vi "AMZ_S3_AUTH_Create HTTP Handle.vi"(4 "Use HTTPS?":bool, 6 "HTTP-Verb":string(combo)="GET", 7 "Redirect endpoint":string, 8 "error in (no error)":errorcluster, 9 "Bucket":string, 10 "Path and query string":string, 11 "Headers":T1[](array[typedef])) -> (0 "error out":errorcluster, 2 "URL":string, 3 "client handle out":T2)   [LabVIEW 2015, in "LV Interface for Amazon S3.lvlib"]
doc: "Create an HTTP Client Handle to Amazon AWS. The handle will hold the necessary Authorozation header which is calculated from many parts and signed with the user's SecretKey."
uses:
  LV Interface for Amazon S3.lvlib
  <vilib>/httpClient/ClientHandle.ctl
  Typedefs/AMZ_S3_HTTP Header-Value pair.ctl
  <vilib>/httpClient/LabVIEWHTTPClient.lvlib
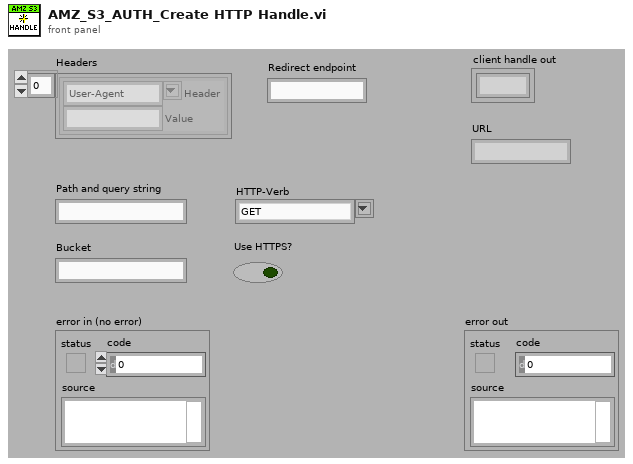
[diagram p1: front panel]
types:
  T1 = typedef "LV Interface for Amazon S3.lvlib/AMZ_S3_HTTP Header-Value pair.ctl" = cluster{"Header":string, "Value":string}
  T2 = typedef "LabVIEWHTTPClient.lvlib/ClientHandle.ctl" = refnum<k1>
  T3 = typedef "LV Interface for Amazon S3.lvlib/AMZ_S3_AWS Credentials.ctl" = cluster{"Access Key":string, "Secret Key":string}
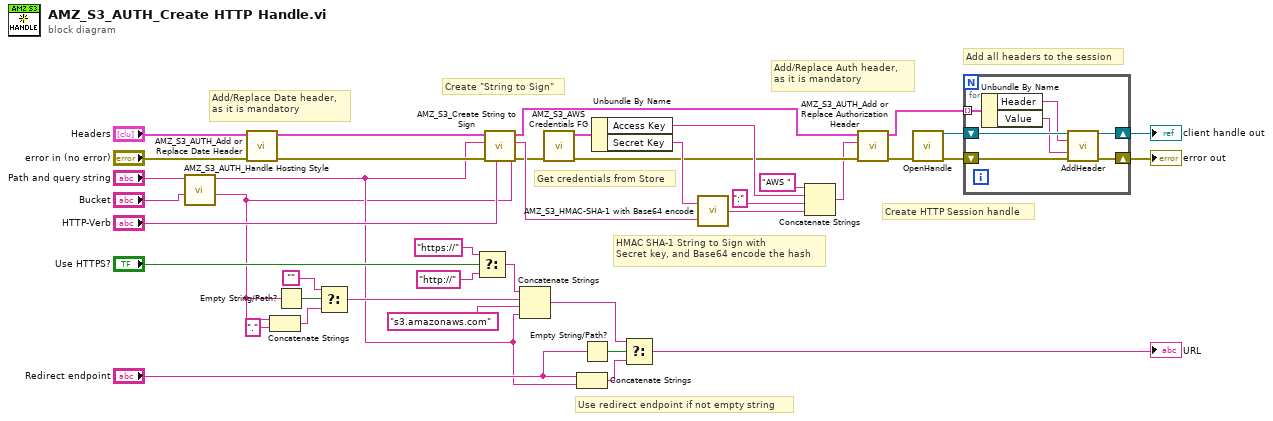
[diagram p0: block diagram]
diagram:
  # "Add all headers to the session"
  # "Create HTTP Session handle"
  # "Add/Replace Auth header,\nas it is mandatory"
  # "HMAC SHA-1 String to Sign with\nSecret key, and Base64 encode the hash"
  # "Get credentials from Store"
  # "Create \"String to Sign\""
  # "Use redirect endpoint if not empty string"
  # "Add/Replace Date header,\nas it is mandatory"
  n1 = call "AMZ_S3_AUTH_Handle Hosting Style.vi"("Bucket in"="Bucket", "Path and query string in"="Path and query string") -> ("Bucket out"=w1:string, "Path and query string out"=w3:string)  [unwired: 8 in]
  n2 = call "AMZ_S3_AUTH_Add or Replace Date Header.vi"("error in (no error)"="error in (no error)", "Headers in"="Headers") -> ("error out"=w21:errorcluster, "Headers"=w22:T1[])  [unwired: 8 in]
  n3 = Concatenate Strings(w1, "." ("string")) -> (w27:string)
  n4 = Empty String/Path?(string/path=w1) -> (empty?=w30:bool)
  n5 = Select(t="", s=w30, f=w27) -> (s? t:f=w26:string)
  n6 = Select(t="https://" ("string"), s="Use HTTPS?", f="http://" ("string")) -> (s? t:f=w6:string)
  n7 = call "AMZ_S3_Create String to Sign.vi"("HTTP-Verb"="HTTP-Verb", "error in (no error)"=w21, "Bucket in"=w1, "Path and query string"=w3, "HTTP Headers in"=w22) -> ("error out"=w20:errorcluster, "StringToSign"=w40:string, "HTTP Headers"=w18:T1[])  [unwired: 4 in]
  n8 = Concatenate Strings(w6, w26, "s3.amazonaws.com" ("string"), w3) -> (w12:string)
  n9 = call "AMZ_S3_AWS Credentials FG.vi"("error in (no error)"=w20) -> ("error out"=w17:errorcluster, "AWS Credentials"=w19:T3)  [unwired: 9 in]
  n10 = Concatenate Strings("Redirect endpoint", w3) -> (w10:string)
  n11 = Empty String/Path?(string/path="Redirect endpoint") -> (empty?=w13:bool)
  n12 = Unbundle By Name(w19) -> ("Access Key"=w35:string, "Secret Key"=w36:string)
  n13 = Select(t=w12, s=w13, f=w10) -> (s? t:f=→"URL":string)
  n14 = call "AMZ_S3_HMAC-SHA-1 with Base64 encode.vi"("Message"=w40, "Key"=w36) -> ("Digest (Base64 encoded)"=w39:string)
  n15 = Concatenate Strings("AWS " ("string"), w35, ":" ("string"), w39) -> (w16:string)
  n16 = call "AMZ_S3_AUTH_Add or Replace Authorization Header.vi"("error in (no error)"=w17, "Authorization Header value"=w16, "Headers in"=w18) -> ("error out"=w15:errorcluster, "Headers"=w14:T1[])  [unwired: 7 in]
  n17 = call <vilib>:"OpenHandle.vi"("error in (no error)"=w15) -> ("client handle out"=w33:T2, "error out"=w34:errorcluster)  [unwired: 13 in]
  n18 = for {
    shift-right: [w46] -> w31
    shift-left: w34 -> [w48]
    shift-right: [w45] -> w32
    shift-left: w33 -> [w47]
    tunnel: w14 -> [w44] mode=indexing
    n19 = Unbundle By Name(w44) -> ("Header"=w43:string, "Value"=w42:string)
    n20 = call <vilib>:"AddHeader.vi"("client handle"=w47, "header"=w43, "value"=w42, "error in (no error)"=w48) -> ("client handle out"=w45:T2, "error out"=w46:errorcluster)  [unwired: 10 in]
  }
  "client handle out" <- w32
  "error out" <- w31
